vi "rs3 delete3.vi"(8 "error in (no error)":errorcluster, 11 "device":u64) -> (0 "error out":errorcluster)   [LabVIEW 2023]
doc: "Delete the device after the sensor has been stopped, closed, deleted."
panel:
  # "RS3 Delete Device"
  # "(C) Intel Corp. 2017, AGJ"
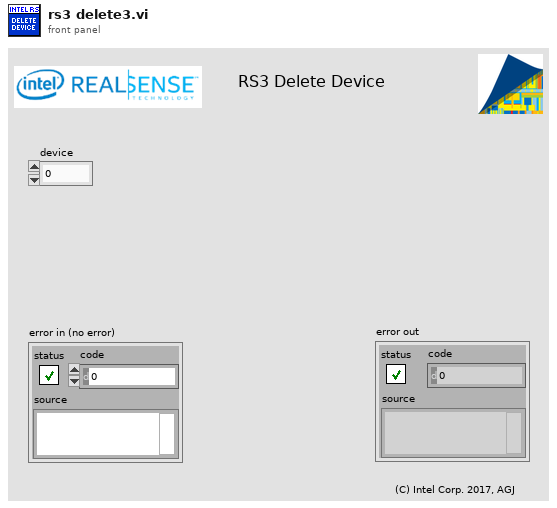
[diagram p1: front panel]
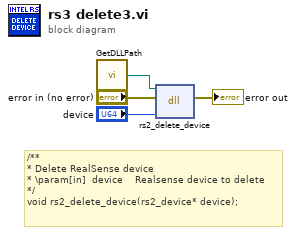
[diagram p0: block diagram]
diagram:
  # "/**\n* Delete RealSense device\n* \\param[in]  device    Realsense device to delete\n*/\nvoid rs2_delete_device(rs2_device* device);"
  n1 = call "GetDLLPath.vi"() -> ("DLL Path"=w1:path)
  n2 = dll-call lib="C:/STEAMSyndicate/RealSenseWrappers/VI Wrappers (add ons) Public/RealSense/realsense2.dll" fn="rs2_delete_device"(path in=w1, error in="error in (no error)", "device"="device") -> (error out=→"error out":errorcluster)  [unwired: 3 in, 1 out]
